vi "Query Instrument Temperature.vi"(8 "error in (no error)":errorcluster, 11 "Manual PSU in":refnum<class "Manual PSU.lvclass">) -> (0 "error out":errorcluster, 2 "Temperature":dbl, 3 "Manual PSU out":refnum<class "Manual PSU.lvclass">)   [LabVIEW 2020, in "Manual PSU.lvclass"]
uses:
  Manual PSU.lvclass
  Power Supply.lvclass
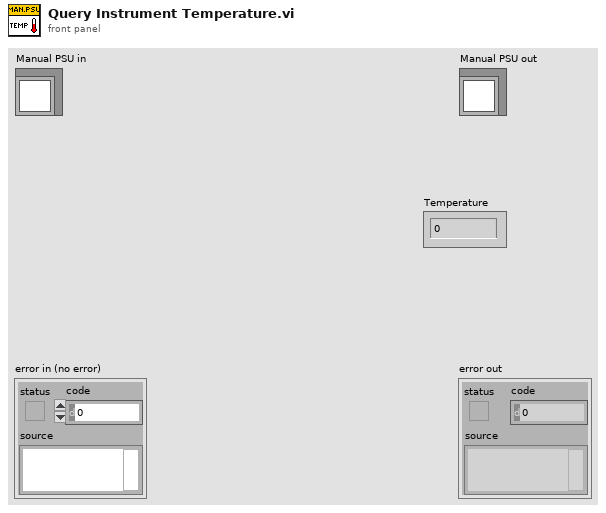
[diagram p1: front panel]
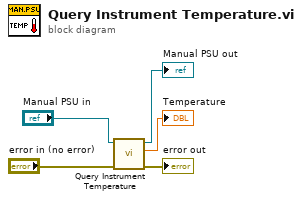
[diagram p0: block diagram]
diagram:
  n1 = call-parent "Query Instrument Temperature.vi"("error in (no error)"="error in (no error)", "Instrument in"="Manual PSU in") -> ("error out"=→"error out":errorcluster, "Temperature"=→"Temperature":dbl, "Instrument out"=→"Manual PSU out":refnum<class "Manual PSU.lvclass">)  [unwired: 7 in]
